vi "aim position.vi"(7 "height":dbl, 8 "velocity":dbl, 9 "distance":dbl) -> (0 "angle":dbl, 3 "distance":dbl)   [LabVIEW 2015]
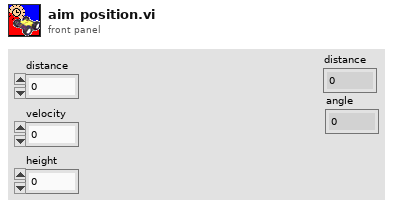
[diagram p1: front panel]
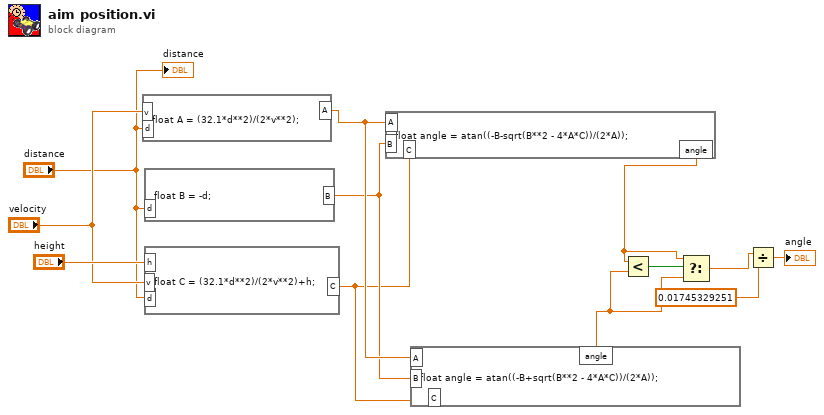
[diagram p0: block diagram]
diagram:
  n1 = formula code="float A = (32.1*d**2)/(2*v**2);"("d"="distance", "v"="velocity") -> ("A"=w10:dbl)
  n2 = formula code="float B = -d;"("d"="distance") -> ("B"=w9:dbl)
  n3 = formula code="float C = (32.1*d**2)/(2*v**2)+h;"("d"="distance", "v"="velocity", "h"="height") -> ("C"=w8:dbl)
  n4 = formula code="float angle = atan((-B-sqrt(B**2 - 4*A*C))/(2*A));"("A"=w10, "B"=w9, "C"=w8) -> ("angle"=w2:dbl)
  n5 = formula code="float angle = atan((-B+sqrt(B**2 - 4*A*C))/(2*A));"("A"=w10, "B"=w9, "C"=w8) -> ("angle"=w6:dbl)
  n6 = Less?(x=w2, y=w6) -> (x < y?=w3:bool)
  n7 = Select(t=w2, s=w3, f=w6) -> (s? t:f=w5:dbl)
  n8 = Divide(x=w5, y=0.01745329251) -> (x/y=→"angle":dbl)
  "distance" <- "distance"
